vi "SubstractDarkPicture.vi"(1 "Dark Pictures":dbl[][][](array[numeric]), 2 "Input":dbl[][](array[numeric]), 4 "Loop index":dbl) -> (5 "Output":dbl[][](array[numeric]))   [LabVIEW 2010]
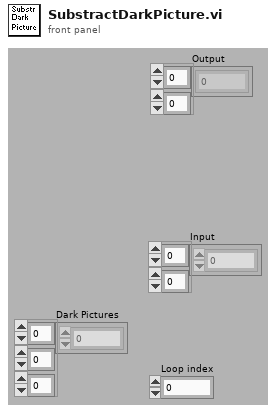
[diagram p1: front panel]
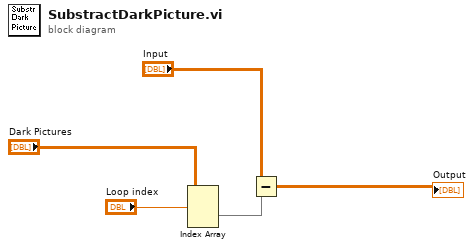
[diagram p0: block diagram]
diagram:
  n1 = Index Array(array="Dark Pictures", index (dim 0)="Loop index") -> (element=w1:dbl[][])  [unwired: 2 in]
  n2 = Subtract(x="Input", y=w1) -> (x-y=→"Output":dbl[][])
